vi "Interpolate 2D Scattered_Cubic.vi"(0 "X":dbl[](array[numeric]), 5 "Y":dbl[](array[numeric]), 7 "Z":dbl[](array[numeric]), 9 "Xi":dbl[](array[numeric]), 11 "Yi":dbl[](array[numeric])) -> (4 "Zi":dbl[](array[numeric]), 15 "error":i32)   [LabVIEW 2017, in "NI_AAL_Interpolation.lvlib"]
uses:
  <vilib>/gmath/NI_AAL_Interpolation.lvlib
  <vilib>/Analysis/NI_AAL_Geometry.lvlib
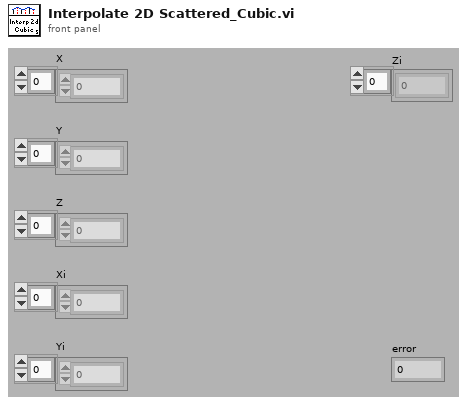
[diagram p1: front panel]
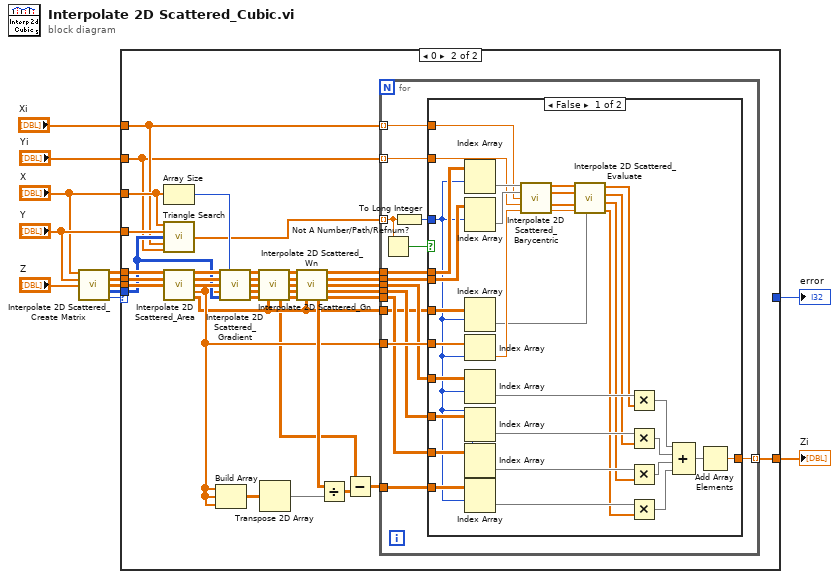
[diagram p0: block diagram]
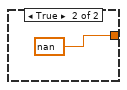
[diagram p3: hidden frame]
diagram:
  n1 = call <vilib>:"Interpolate 2D Scattered_Create Matrix.vi"("X"="X", "Y"="Y", "Z"="Z") -> ("X(Tri)"=w10:dbl[][], "Y(Tri)"=w9:dbl[][], "Z(Tri)"=w8:dbl[][], "Triangles"=w7:i32[][], "error"=w2:i32)  [unwired: 8 out]
  n2 = case shown="0" w2 {
    selector: w2 -> [w13 _]
    tunnel: "Y" -> [_ w50]
    tunnel: w10 -> [_ w49]
    tunnel: w9 -> [_ w48]
    tunnel: w8 -> [_ w47]
    tunnel: w7 -> [_ w43]
    tunnel: "X" -> [_ w42]
    tunnel: "Xi" -> [_ w15]
    tunnel: "Yi" -> [_ w14]
    tunnel: [_ w16] -> w3
    tunnel: [w13 _] -> w1
    frame -1, Default {
    }
    frame 0 {
      n3 = Array Size(array=w42) -> (size(s)=w41:i32)
      n4 = call <vilib>:"Triangle Search.vi"("X"=w42, "Y"=w50, "Triangles"=w43, "Xi"=w15, "Yi"=w14) -> ("indices"=w27:dbl[])  [unwired: 10 out]
      n5 = call <vilib>:"Interpolate 2D Scattered_Area.vi"("X(Tri) In"=w49, "Y(Tri) In"=w48, "Z(Tri)  In"=w47) -> ("X(Tri) Out"=w46:dbl[][], "Y(Tri) Out"=w45:dbl[][], "Z(Tri) Out"=w44:dbl[][], "Area"=w21:dbl[], "Length"=w20:dbl[][])  [unwired: 8 out]
      n6 = Build Array(w21, w21, w21) -> (w30:dbl[][])
      n7 = call <vilib>:"Interpolate 2D Scattered_Gradient.vi"("X(Tri) In"=w46, "point number"=w41, "Y(Tri) In"=w45, "Z(Tri) In"=w44, "Area"=w21, "Triangles"=w43) -> ("X(Tri) Out"=w40:dbl[][], "Y(Tri) Out"=w39:dbl[][], "Z(Tri) Out"=w38:dbl[][], "gx"=w37:dbl[][], "gy"=w36:dbl[][])  [unwired: 5 out]
      n8 = call <vilib>:"Interpolate 2D Scattered_Gn.vi"("X(Tri) In"=w40, "Y(Tri) In"=w39, "Z(Tri) In"=w38, "gx in"=w37, "gy in"=w36, "Length"=w20) -> ("X(Tri) Out"=w35:dbl[][], "Y(Tri) Out"=w34:dbl[][], "Z(Tri) Out"=w33:dbl[][], "gx out"=w32:dbl[][], "Gn"=w18:dbl[][], "gy out"=w31:dbl[][])  [unwired: 4 out]
      n9 = Transpose 2D Array(2D array=w30) -> (transposed array=w29:dbl[][])
      n10 = call <vilib>:"Interpolate 2D Scattered_Wn.vi"("X(Tri) In"=w35, "Y(Tri) In"=w34, "Z(Tri) In"=w33, "gx in"=w32, "gy in"=w31, "Length"=w20) -> ("X(Tri) Out"=w26:dbl[][], "Y(Tri) Out"=w25:dbl[][], "Z(Tri) Out"=w24:dbl[][], "gx out"=w23:dbl[][], "Wn"=w28:dbl[][], "gy out"=w22:dbl[][])  [unwired: 4 in]
      n11 = Divide(x=w28, y=w29) -> (x/y=w19:dbl[][])
      n12 = Subtract(x=w18, y=w19) -> (x-y=w17:dbl[][])
      n13 = for {
        tunnel: w27 -> [w63] mode=indexing
        tunnel: w15 -> [w62] mode=indexing
        tunnel: w14 -> [w61] mode=indexing
        tunnel: w26 -> [w59]
        tunnel: w25 -> [w58]
        tunnel: w24 -> [w57]
        tunnel: w23 -> [w56]
        tunnel: w22 -> [w55]
        tunnel: w21 -> [w60]
        tunnel: w20 -> [w54]
        tunnel: w17 -> [w52]
        tunnel: [w51] -> w16 mode=indexing
        n14 = Not A Number/Path/Refnum?(number/path/refnum=w63) -> (NaN/Path/Refnum?=w64:bool)
        n15 = To Long Integer(number=w63) -> (32bit integer=w53:i32)
        n16 = case shown="False" w64 {
          tunnel: w53 -> [w84 _]
          tunnel: w62 -> [w92 _]
          tunnel: w61 -> [w91 _]
          tunnel: w60 -> [w95 _]
          tunnel: w59 -> [w97 _]
          tunnel: w58 -> [w96 _]
          tunnel: w57 -> [w86 _]
          tunnel: w56 -> [w87 _]
          tunnel: w55 -> [w88 _]
          tunnel: w54 -> [w85 _]
          tunnel: w52 -> [w89 _]
          tunnel: [w67 nan] -> w51
          frame False {
            n17 = Index Array(array=w97, index (row)=w84) -> (element=w94:dbl[])  [unwired: 1 in]
            n18 = Index Array(array=w96, index (row)=w84) -> (element=w93:dbl[])  [unwired: 1 in]
            n19 = Index Array(array=w85, index (row)=w84) -> (element=w81:dbl[])  [unwired: 1 in]
            n20 = Index Array(array=w95, index=w84) -> (element=w90:dbl)
            n21 = Index Array(array=w86, index (row)=w84) -> (element=w78:dbl[])  [unwired: 1 in]
            n22 = Index Array(array=w87, index (row)=w84) -> (element=w76:dbl[])  [unwired: 1 in]
            n23 = Index Array(array=w88, index (row)=w84) -> (element=w74:dbl[])  [unwired: 1 in]
            n24 = Index Array(array=w89, index (row)=w84) -> (element=w72:dbl[])  [unwired: 1 in]
            n25 = call <vilib>:"Interpolate 2D Scattered_Barycentric.vi"("X In"=w94, "Y In"=w93, "x"=w92, "y"=w91, "area in"=w90) -> ("X Out"=w83:dbl[], "Y Out"=w82:dbl[], "W"=w79:dbl[], "area out"=w80:dbl)  [unwired: 7 out]
            n26 = call <vilib>:"Interpolate 2D Scattered_Evaluate.vi"("Length"=w81, "area"=w80, "W"=w79, "Y"=w82, "X"=w83) -> ("M"=w71:dbl[], "N3"=w73:dbl[], "N2"=w75:dbl[], "N1"=w77:dbl[])  [unwired: 3 in]
            n27 = Multiply(x=w78, y=w77) -> (x*y=w69:dbl[])
            n28 = Multiply(x=w76, y=w75) -> (x*y=w70:dbl[])
            n29 = Multiply(x=w74, y=w73) -> (x*y=w65:dbl[])
            n30 = Multiply(x=w72, y=w71) -> (x*y=w66:dbl[])
            n31 = Compound Arithmetic op=ADD(w69, w70, w65, w66) -> (w68:dbl[])
            n32 = Add Array Elements(numeric array=w68) -> (sum=w67:dbl)
          }
          frame True {
          }
        }
      }
    }
  }
  "Zi" <- w3
  "error" <- w1
